vi "ControlMotorFindZeroAll.vi"(8 "错误输入":errorcluster caption="错误常量") -> (0 "error IO":errorcluster)   [LabVIEW 2018]
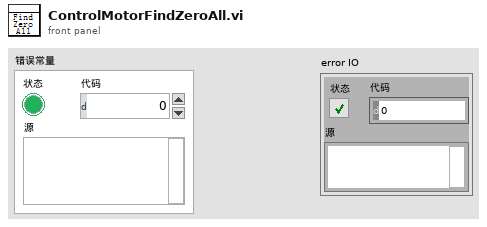
[diagram p1: front panel]
types:
  T1 = typedef "控制电机枚举器.ctl" = enum16{"Z", "Y", "X", "发散角", "俯仰", "旋转"}
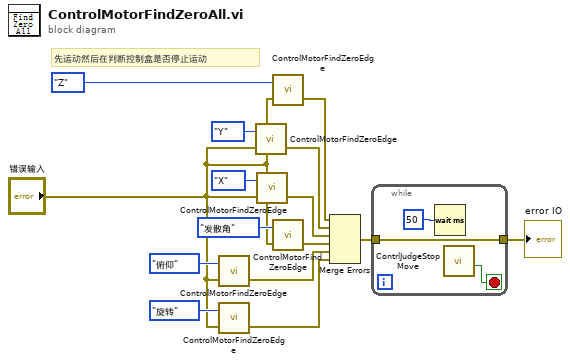
[diagram p0: block diagram]
diagram:
  # "先运动然后在判断控制盒是否停止运动"
  n1 = call "ControlMotorFindZeroEdge.vi"("错误输入"="错误输入", "控制电机"=控制电机枚举器."俯仰") -> ("错误输出"=w8:errorcluster)  [unwired: 1 in]
  n2 = call "ControlMotorFindZeroEdge.vi"("错误输入"="错误输入", "控制电机"=控制电机枚举器."旋转") -> ("错误输出"=w4:errorcluster)  [unwired: 1 in]
  n3 = call "ControlMotorFindZeroEdge.vi"("错误输入"="错误输入", "控制电机"=控制电机枚举器."Y") -> ("错误输出"=w7:errorcluster)  [unwired: 1 in]
  n4 = call "ControlMotorFindZeroEdge.vi"("错误输入"="错误输入", "控制电机"=控制电机枚举器."X") -> ("错误输出"=w6:errorcluster)  [unwired: 1 in]
  n5 = call "ControlMotorFindZeroEdge.vi"("错误输入"="错误输入", "控制电机"=控制电机枚举器."Z") -> ("错误输出"=w10:errorcluster)  [unwired: 1 in]
  n6 = call "ControlMotorFindZeroEdge.vi"("错误输入"="错误输入", "控制电机"=控制电机枚举器."发散角") -> ("错误输出"=w9:errorcluster)  [unwired: 1 in]
  n7 = Merge Errors(w10, w7, w6, w9, w8, w4) -> (w3:errorcluster)
  n8 = while {
    tunnel: w3 -> [w17]
    tunnel: [w17] -> w1
    stop <- w16 stop-if-true
    n9 = Wait (ms)(milliseconds to wait=u32 50 ("等待时间（毫秒）")) -> ()  [unwired: 1 out]
    n10 = call "ContrlJudgeStopMove.vi"() -> ("是否停止运动？"=w16:bool)  [unwired: 11 in]
  }
  "error IO" <- w1
